vi "WlArraySplitter.vi"(2 "Cutoff Wavelength":dbl=700.0 format="%#_13g", 3 "Wavelength Array":dbl[](array[numeric])) -> (0 "Higher Wavelengths":dbl[](array[numeric]), 1 "Lower Wavelengths":dbl[](array[numeric]))   [LabVIEW 2018]
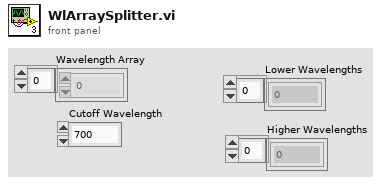
[diagram p1: front panel]
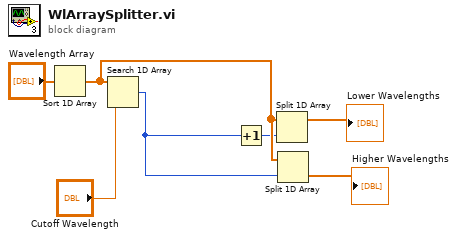
[diagram p0: block diagram]
diagram:
  n1 = Sort 1D Array(array="Wavelength Array") -> (sorted array=w5:dbl[])
  n2 = Search 1D Array(1D array=w5, element="Cutoff Wavelength") -> (index of element=w6:i32)  [unwired: 1 in]
  n3 = Increment(x=w6) -> (x+1=w4:i32)
  n4 = Split 1D Array(array=w5, index=w4) -> (first subarray=→"Lower Wavelengths":dbl[])  [unwired: 1 out]
  n5 = Split 1D Array(array=w5, index=w6) -> (second subarray=→"Higher Wavelengths":dbl[])  [unwired: 1 out]
